vi "DEPP Write Read.vi"() -> ()   [LabVIEW 2011, in "LVH-Adept.lvlib"]
uses:
  LVH-Adept.lvlib
  Private/DMGR/DMGR.lvlib
  Private/DEPP/DEPP.lvlib
panel:
  out "Data 2":u8
  in  "Data":u8
  in  "Address":u8
  out "Error Out":errorcluster
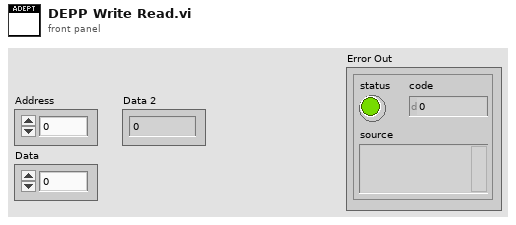
[diagram p1: front panel]
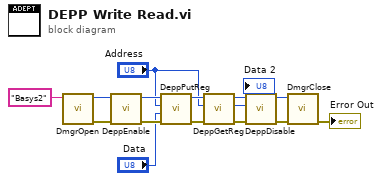
[diagram p0: block diagram]
diagram:
  n1 = call "DmgrOpen.vi"("Device Name"="Basys2") -> ("Error Out"=w15:errorcluster, "Device Handle"=w12:u32)  [unwired: 9 in]
  n2 = call "DeppEnable.vi"("Error In"=w15, "Device Handle"=w12) -> ("Error Out"=w8:errorcluster, "Device Handle"=w9:u32)  [unwired: 8 in]
  n3 = call "DeppPutReg.vi"("Error In"=w8, "Data"="Data", "Address"="Address", "Device Handle"=w9) -> ("Error Out"=w7:errorcluster, "Device Handle"=w4:u32)  [unwired: 6 in]
  n4 = call "DeppGetReg.vi"("Error In"=w7, "Address"="Address", "Device Handle"=w4) -> ("Error Out"=w6:errorcluster, "Data"=→"Data 2":u8, "Device Handle"=w5:u32)  [unwired: 6 in]
  n5 = call "DeppDisable.vi"("Error In"=w6, "Device Handle"=w5) -> ("Error Out"=w14:errorcluster, "Device Handle"=w13:u32)  [unwired: 8 in]
  n6 = call "DmgrClose.vi"("Error In"=w14, "hif"=w13) -> ("Error Out"=→"Error Out":errorcluster)  [unwired: 9 in]
